vi "String Functions (SubVI).vi"(7 "String Function":T1=enum."Build Primary", 8 "error in":errorcluster, 11 "Function String":string) -> (0 "error out":errorcluster, 2 "Secondary Display String":string, 3 "Primary Display String":string)   [LabVIEW 2012]
doc: "Performs all the string operations for both Primary and Secondary strings. The function is controlled by the String Function enum, which is defined by String Commands.ctl"
uses:
  Controls/String Commands.ctl
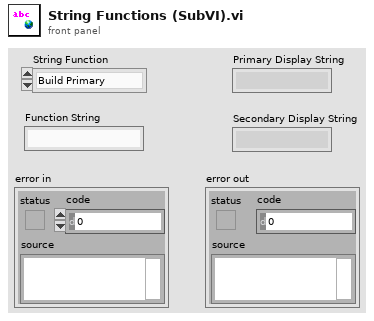
[diagram p1: front panel]
types:
  T1 = typedef "String Commands.ctl" = enum16{"GET Strings", "Set Secondary", "Build Primary", "Build Secondary", "Backspace", "Replace Operator", "Clear Primary", "Clear Secondary", "Clear ALL", "Decimal Point"}
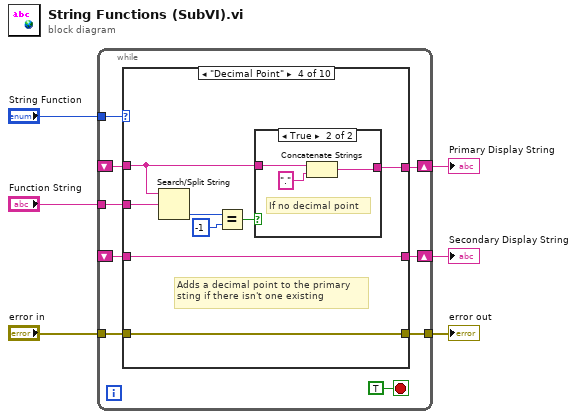
[diagram p0: block diagram]
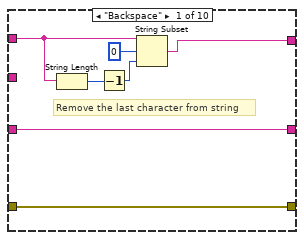
[diagram p2: hidden frame]
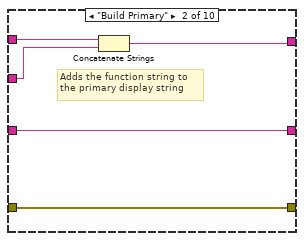
[diagram p3: hidden frame]
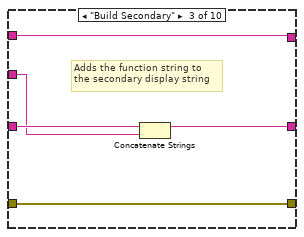
[diagram p4: hidden frame]
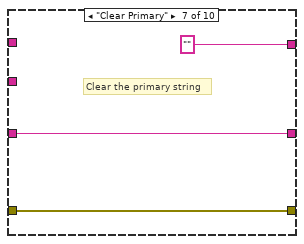
[diagram p8: hidden frame]
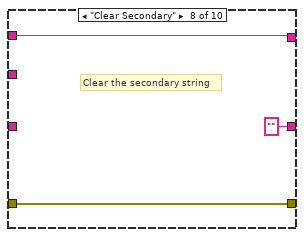
[diagram p9: hidden frame]
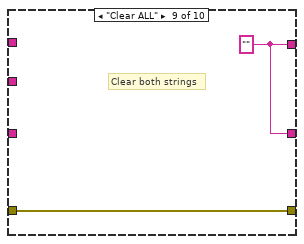
[diagram p10: hidden frame]
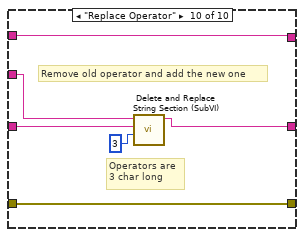
[diagram p11: hidden frame]
diagram:
  n1 = while {
    tunnel: "String Function" -> [w14]
    shift-right: [w13] -> w5
    shift-left: _ -> [w15]
    tunnel: "Function String" -> [w11]
    tunnel: "error in" -> [w10]
    tunnel: [w9] -> w2
    shift-right: [w7] -> w1
    shift-left: _ -> [w8]
    stop <- TRUE stop-if-true
    n2 = case shown="\"Decimal Point\"" w14 {
      tunnel: w15 -> [w21 w26 w28 w35 w45 w49 _ w55 _ w63]
      tunnel: [w18 w27 w28 w34 w45 w49 "" w55 w56 w63] -> w13
      tunnel: w11 -> [_ w25 w30 w39 _ _ _ _ _ w59]
      tunnel: w10 -> [w17 w24 w32 w40 w46 w48 w52 w54 w57 w62]
      tunnel: [w17 w24 w32 w40 w46 w48 w52 w54 w57 w62] -> w9
      tunnel: w8 -> [w16 w23 w31 w33 _ w47 w50 _ _ w61]
      tunnel: [w16 w23 w29 w33 w45 w47 w50 "" ("String in") w56 w58] -> w7
      frame "Backspace" {
        # "Remove the last character from string"
        n3 = String Length(string=w21) -> (length=w22:i32)
        n4 = Decrement(x=w22) -> (x-1=w20:i32)
        n5 = String Subset(string=w21, offset (0)=0, length (rest)=w20) -> (substring=w18:string)
      }
      frame "Build Primary" {
        # "Adds the function string to\nthe primary display string"
        n6 = Concatenate Strings(w26, w25) -> (w27:string)
      }
      frame "Build Secondary" {
        # "Adds the function string to\nthe secondary display string"
        n7 = Concatenate Strings(w31, w30) -> (w29:string)
      }
      frame "Decimal Point" {
        # "Adds a decimal point to the primary\nsting if there isn't one existing"
        n8 = Search/Split String(string=w35, search string/char (-)=w39) -> (offset of match=w38:i32)  [unwired: 1 in, 2 out]
        n9 = Equal?(x=w38, y=-1) -> (x = y?=w36:bool)
        n10 = case shown="True" w36 {
          tunnel: w35 -> [w41 w44]
          tunnel: [w41 w42] -> w34
          frame False {
            # "Ignore if decimal\nalready there"
          }
          frame True {
            # "If no decimal point"
            n11 = Concatenate Strings(w44, "." ("string")) -> (w42:string)
          }
        }
      }
      frame "Set Secondary" {
        # "Set the secondary string to be the\nsame as the current primary string"
      }
      frame "GET Strings" {
        # "Return the Primary and Secondary\nstrings stored in the shift registers"
      }
      frame "Clear Primary" {
        # "Clear the primary string"
      }
      frame "Clear Secondary" {
        # "Clear the secondary string"
      }
      frame "Clear ALL" {
        w56 = "" ("String in")
        # "Clear both strings"
      }
      frame "Replace Operator" {
        # "Remove old operator and add the new one"
        # "Operators are \n3 char long"
        n12 = call "Delete and Replace String Section (SubVI).vi"("Length"=3 ("y"), "Secondary String In"=w61, "Function String"=w59) -> ("Secondary String Out"=w58:string)  [unwired: 8 in]
      }
    }
  }
  "Primary Display String" <- w5
  "error out" <- w2
  "Secondary Display String" <- w1
